vi "Begin.vi"(8 "error in":errorcluster) -> (0 "error out":errorcluster)   [LabVIEW 2016]
doc: "Called before other user functions, this VI is expected to open initial I/O refnums, load in file data, and do all program initialization. Notice that the <B>error out</B> terminal is simply used for data flow. Wiring it to other structures or subVIs ensures that this VI runs first."
uses:
  <vilib>/Rock Robotics/WPI/DriverStation/WPI_DriverStationRobotMode2.ctl
  <vilib>/Rock Robotics/SystemInterfaces/DIO/FPGA_DIOPWMChannel.ctl
  <vilib>/Rock Robotics/WPI/Joystick/WPI_JoystickDeviceEnum.ctl
  <vilib>/Rock Robotics/WPI/Solenoid/WPI_SolenoidChannel.ctl
  <vilib>/Rock Robotics/WPI/Camera/WPI_CameraExposure Values.ctl
  <vilib>/Rock Robotics/WPI/Camera/WPI_CameraWhite Balance Values.ctl
  <vilib>/Rock Robotics/WPI/Camera/WPI_CameraFrameRate.ctl
  <vilib>/Rock Robotics/WPI/Camera/WPI_CameraImageSize.ctl
  <vilib>/Rock Robotics/SystemInterfaces/DIO/FPGA_DIOChannel.ctl
  SubSystems/References/CameraDevRef 0.vi
  <vilib>/Rock Robotics/Network Tables/NT Write String Array.vi
  <vilib>/Rock Robotics/WPI/MotorControl/WPI_MotorControlOpen Talon.vi
  <vilib>/Rock Robotics/WPI/Solenoid/WPI_SolenoidOpenDouble.vi
  SubSystems/References/Refnums.vi
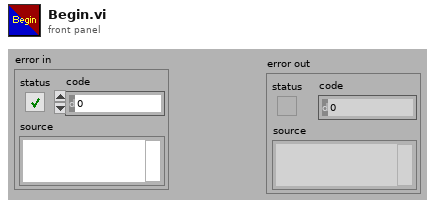
[diagram p1: front panel]
types:
  T1 = typedef "FPGA_DIOChannel.ctl" = enum8{"DIO 0", "DIO 1", "DIO 2", "DIO 3", "DIO 4", "DIO 5", "DIO 6", "DIO 7", "DIO 8", "DIO 9", "DIO MXP 0", "DIO MXP 1", "DIO MXP 2", "DIO MXP 3", "DIO MXP 4", "DIO MXP 5", "DIO MXP 6", "DIO MXP 7", "DIO MXP 8", "DIO MXP 9", "DIO MXP 10", "DIO MXP 11", "DIO MXP 12", "DIO MXP 13", "DIO MXP 14", "DIO MXP 15", "SPI Port CS1", "SPI Port CS2", "SPI Port CS3", "SPI Port MISO", "SPI Port MOSI", "Invalid"}
  T2 = typedef "WPI_CameraImageSize.ctl" = enum16{"640x480", "320x240", "160x120", "Custom"}
  T3 = typedef "WPI_CameraFrameRate.ctl" = u32
  T4 = typedef "WPI_CameraExposure Values.ctl" = enum16{"Auto", "Flicker-free 50 Hz", "Flicker-free 60 Hz", "Hold current", "Custom"}
  T5 = typedef "WPI_CameraWhite Balance Values.ctl" = enum16{"Auto", "Fixed indoor", "Fixed outdoor 1", "Fixed outdoor 2", "Fixed fluorescent 1", "Fixed fluorescent 2", "Hold current", "Custom"}
  T6 = typedef "FPGA_DIOPWMChannel.ctl" = enum8{"PWM 0", "PWM 1", "PWM 2", "PWM 3", "PWM 4", "PWM 5", "PWM 6", "PWM 7", "PWM 8", "PWM 9", "PWM MXP 0", "PWM MXP 1", "PWM MXP 2", "PWM MXP 3", "PWM MXP 4", "PWM MXP 5", "PWM MXP 6", "PWM MXP 7", "PWM MXP 8", "PWM MXP 9", "Invalid"}
  T7 = typedef "WPI_SolenoidChannel.ctl" = enum8{"Solenoid 0", "Solenoid 1", "Solenoid 2", "Solenoid 3", "Solenoid 4", "Solenoid 5", "Solenoid 6", "Solenoid 7", "Invalid"}
  T8 = typedef "WPI_JoystickDeviceEnum.ctl" = enum16{"USB 0", "USB 1", "USB 2", "USB 3", "USB 4", "USB 5"}
  T9 = typedef "WPI_DriverStationRobotMode2.ctl" = enum16{"Autonomous Disabled", "Autonomous Enabled", "Teleop Disabled", "Teleop Enabled", "Disconnected", "Finish", "Test Disabled", "Test Enabled", "Emergency Stopped"}
  T10 = typedef "WPI_CameraDevRef.ctl" = cluster{"Camera Address":string, "CameraStatus":errorcluster}
  T11 = typedef "WPI_JoystickDevRef.ctl" = cluster{"Device":T8}
  T12 = typedef "WPI_MotorControlDeviceRef.ctl" = cluster{"DeviceStatus":errorcluster, "Type":T13, "PWM":cluster{"PWM Channel":T6, "DeadBand":T14}, "CAN":cluster{"Device Number":u8, "SetOutput VI Ref":variant, "GetOutput VI Ref":variant, "Enable VI Ref":variant, "Disable VI Ref":variant, "Data":variant}, "Invert":bool}
  T13 = typedef "WPI_MotorControlType.ctl" = enum16{"PWM", "CAN"}
  T14 = typedef "WPI_PWMDeadband.ctl" = cluster{"Name":string, "maxPositivePwm":i32, "minPositivePwm":i32, "centerPwm":i32, "maxNegativePwm":i32, "minNegativePwm":i32, "angularRange":u16}
  T15 = typedef "WPI_DigitalInputDevRef.ctl" = cluster{"DevStatus":errorcluster, "DIO Channel":T1}
  T16 = typedef "WPI_SolenoidDevRef.ctl" = cluster{"DevStatus":errorcluster, "Pneumatics Control Module":u8, "Forward Solenoid Channel":T7, "Reverse Solenoid Channel":T7}
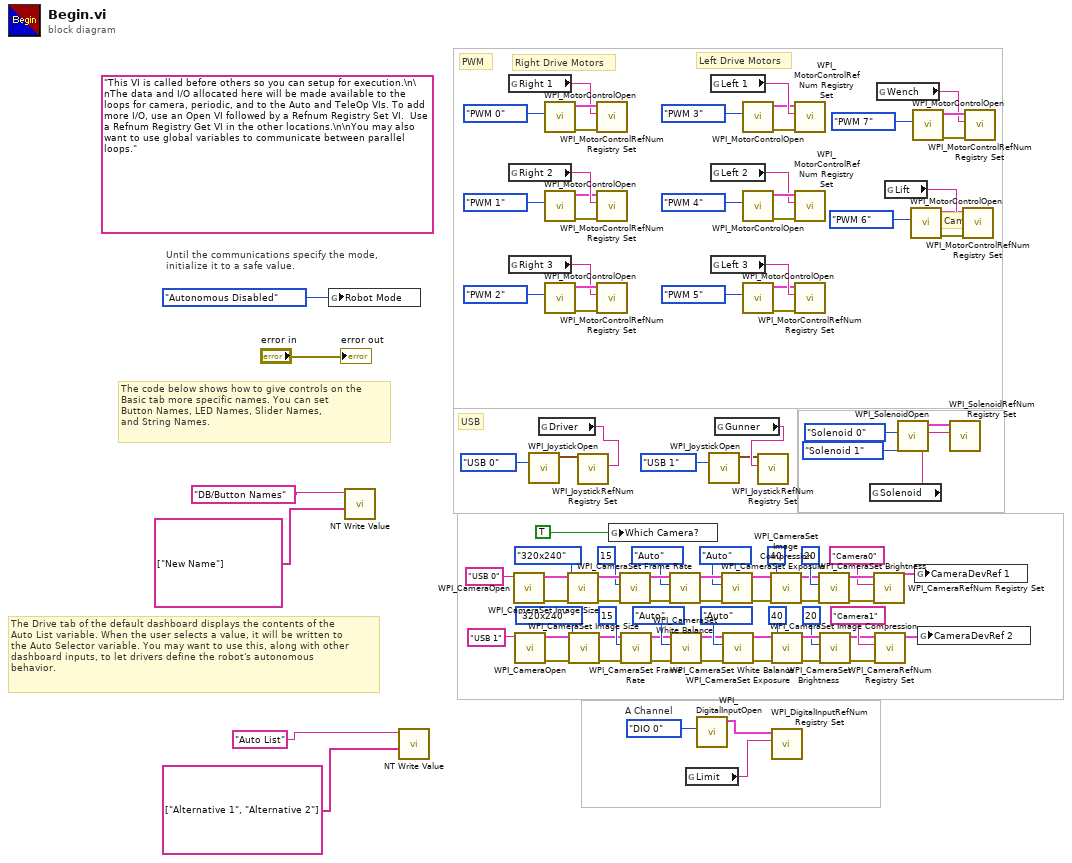
[diagram p0: block diagram]
diagram:
  w3 = FPGA_DIOChannel."DIO 0"  # A Channel
  (unwired) "This VI is called before others so you can setup for execution.\n\nThe data and I/O allocated here will be made available to the loops for camera, periodic, and to the Auto and TeleOp VIs. To add more I/O, use an Open VI followed by a Refnum Registry Set VI.  Use a Refnum Registry Get VI in the other locations.\n\nYou may also want to use global variables to communicate between parallel loops."
  # "Cameras"
  # "USB"
  # "Left Drive Motors"
  # "Right Drive Motors"
  # "PWM"
  # "The Drive tab of the default dashboard displays the contents of the\nAuto List variable. When the user selects a value, it will be written to\nthe Auto Selector variable. You may want to use this, along with other\ndashboard inputs, to let drivers define the robot's autonomous\nbehavior."
  # "The code below shows how to give controls on the\nBasic tab more specific names. You can set\nButton Names, LED Names, Slider Names,\nand String Names."
  # "Until the communications specify the mode,\ninitialize it to a safe value."
  n1 = global write "CameraDevRef 0.vi" "Robot Mode"(WPI_DriverStationRobotMode2."Autonomous Disabled" ("Robot Mode")) -> ()
  n2 = call-poly <vilib>:"NT Write Value.vi"("String Array"=string[] ["New Name"], "Name"="DB/Button Names") -> ()  [unwired: 9 in, 1 out]
  n3 = call-poly <vilib>:"NT Write Value.vi"("String Array"=string[] ["Alternative 1", "Alternative 2"], "Name"="Auto List") -> ()  [unwired: 9 in, 1 out]
  n4 = global read "Refnums.vi" "Right 1"() -> (w89:string)
  n5 = global read "Refnums.vi" "Right 2"() -> (w88:string)
  n6 = global read "Refnums.vi" "Right 3"() -> (w81:string)
  n7 = call <vilib>:"WPI_CameraOpen.vi"("Camera Address"="USB 0") -> ("error out"=w40:errorcluster, "CameraDevRef"=w41:T10)  [unwired: 1 in, 8 out]
  n8 = call <vilib>:"WPI_CameraOpen.vi"("Camera Address"="USB 1") -> ("error out"=w19:errorcluster, "CameraDevRef"=w18:T10)  [unwired: 1 in, 8 out]
  n9 = call <vilib>:"WPI_JoystickOpen.vi"("JoystickDevice"=WPI_JoystickDeviceEnum."USB 0") -> ("JoystickDevRef"=w64:T11)  [unwired: 10 in]
  n10 = global read "Refnums.vi" "Driver"() -> (w63:string)
  n11 = call-poly <vilib>:"WPI_MotorControlOpen.vi"("PWM Channel"=FPGA_DIOPWMChannel."PWM 0") -> ("error out"=w92:errorcluster, "MotorControlDeviceRef"=w91:T12)  [unwired: 9 in]
  n12 = call-poly <vilib>:"WPI_MotorControlOpen.vi"("PWM Channel"=FPGA_DIOPWMChannel."PWM 1") -> ("error out"=w85:errorcluster, "MotorControlDeviceRef"=w86:T12)  [unwired: 9 in]
  n13 = call-poly <vilib>:"WPI_MotorControlOpen.vi"("PWM Channel"=FPGA_DIOPWMChannel."PWM 2") -> ("error out"=w84:errorcluster, "MotorControlDeviceRef"=w83:T12)  [unwired: 9 in]
  n14 = call <vilib>:"WPI_CameraSet Image Size.vi"("error in (no error)"=w40, "Image Size"=WPI_CameraImageSize."320x240", "CameraDevRef"=w41) -> ("error out"=w39:errorcluster, "CameraDevRef Out"=w42:T10)  [unwired: 1 in, 6 out]
  n15 = call <vilib>:"WPI_CameraSet Image Size.vi"("error in (no error)"=w19, "Image Size"=WPI_CameraImageSize."320x240", "CameraDevRef"=w18) -> ("error out"=w20:errorcluster, "CameraDevRef Out"=w17:T10)  [unwired: 1 in, 6 out]
  n16 = call <vilib>:"WPI_JoystickRefNum Registry Set.vi"("refnum name"=w63, "JoystickDevRef"=w64) -> ()  [unwired: 8 in, 2 out]
  n17 = call <vilib>:"WPI_MotorControlRefNum Registry Set.vi"("error in (no error)"=w92, "refnum name"=w89, "MotorControlDevRef"=w91) -> ()  [unwired: 7 in, 2 out]
  n18 = call <vilib>:"WPI_MotorControlRefNum Registry Set.vi"("error in (no error)"=w85, "refnum name"=w88, "MotorControlDevRef"=w86) -> ()  [unwired: 7 in, 2 out]
  n19 = call <vilib>:"WPI_MotorControlRefNum Registry Set.vi"("error in (no error)"=w84, "refnum name"=w81, "MotorControlDevRef"=w83) -> ()  [unwired: 7 in, 2 out]
  n20 = global write "Refnums.vi" "Which Camera?"(TRUE ("Which Camera?")) -> ()
  n21 = call <vilib>:"WPI_CameraSet Frame Rate.vi"("error in (no error)"=w39, "Frame Rate (fps)"=T3 15, "CameraDevRef"=w42) -> ("error out"=w38:errorcluster, "CameraDevRef Out"=w44:T10)  [unwired: 7 out]
  n22 = call <vilib>:"WPI_CameraSet Frame Rate.vi"("error in (no error)"=w20, "Frame Rate (fps)"=T3 15, "CameraDevRef"=w17) -> ("error out"=w21:errorcluster, "CameraDevRef Out"=w15:T10)  [unwired: 7 out]
  n23 = call <vilib>:"WPI_CameraSet White Balance.vi"("error in (no error)"=w38, "White Balance"=WPI_CameraWhite_Balance_Values."Auto", "CameraDevRef"=w44) -> ("error out"=w37:errorcluster, "CameraDevRef Out"=w43:T10)  [unwired: 1 in, 6 out]
  n24 = call <vilib>:"WPI_CameraSet White Balance.vi"("error in (no error)"=w21, "White Balance"=WPI_CameraWhite_Balance_Values."Auto", "CameraDevRef"=w15) -> ("error out"=w22:errorcluster, "CameraDevRef Out"=w16:T10)  [unwired: 1 in, 6 out]
  n25 = global read "Refnums.vi" "Limit"() -> (w1:string)
  n26 = call <vilib>:"WPI_DigitalInputOpen.vi"("DIO Channel"=w3) -> ("DigitalInputDevRef"=w2:T15)  [unwired: 1 in, 9 out]
  n27 = call <vilib>:"WPI_JoystickOpen.vi"("JoystickDevice"=WPI_JoystickDeviceEnum."USB 1") -> ("JoystickDevRef"=w59:T11)  [unwired: 10 in]
  n28 = global read "Refnums.vi" "Left 1"() -> (w72:string)
  n29 = global read "Refnums.vi" "Left 2"() -> (w73:string)
  n30 = global read "Refnums.vi" "Left 3"() -> (w80:string)
  n31 = global read "Refnums.vi" "Gunner"() -> (w60:string)
  n32 = call <vilib>:"WPI_CameraSet Exposure.vi"("error in (no error)"=w37, "Exposure"=WPI_CameraExposure_Values."Auto", "CameraDevRef"=w43) -> ("error out"=w36:errorcluster, "CameraDevRef Out"=w46:T10)  [unwired: 1 in, 6 out]
  n33 = call <vilib>:"WPI_CameraSet Exposure.vi"("error in (no error)"=w22, "Exposure"=WPI_CameraExposure_Values."Auto", "CameraDevRef"=w16) -> ("error out"=w23:errorcluster, "CameraDevRef Out"=w13:T10)  [unwired: 1 in, 6 out]
  n34 = call-poly <vilib>:"WPI_MotorControlOpen.vi"("PWM Channel"=FPGA_DIOPWMChannel."PWM 3") -> ("error out"=w69:errorcluster, "MotorControlDeviceRef"=w70:T12)  [unwired: 9 in]
  n35 = call-poly <vilib>:"WPI_MotorControlOpen.vi"("PWM Channel"=FPGA_DIOPWMChannel."PWM 4") -> ("error out"=w76:errorcluster, "MotorControlDeviceRef"=w75:T12)  [unwired: 9 in]
  n36 = call-poly <vilib>:"WPI_MotorControlOpen.vi"("PWM Channel"=FPGA_DIOPWMChannel."PWM 5") -> ("error out"=w77:errorcluster, "MotorControlDeviceRef"=w78:T12)  [unwired: 9 in]
  n37 = call <vilib>:"WPI_JoystickRefNum Registry Set.vi"("refnum name"=w60, "JoystickDevRef"=w59) -> ()  [unwired: 8 in, 2 out]
  n38 = call <vilib>:"WPI_CameraSet Image Compression.vi"("error in (no error)"=w36, "Compression"=40, "CameraDevRef"=w46) -> ("error out"=w35:errorcluster, "CameraDevRef Out"=w45:T10)  [unwired: 7 out]
  n39 = call <vilib>:"WPI_CameraSet Image Compression.vi"("error in (no error)"=w23, "Compression"=40, "CameraDevRef"=w13) -> ("error out"=w24:errorcluster, "CameraDevRef Out"=w14:T10)  [unwired: 7 out]
  n40 = call <vilib>:"WPI_DigitalInputRefNum Registry Set.vi"("refnum name"=w1, "DigitalInputDevRef"=w2) -> ()  [unwired: 8 in, 2 out]
  n41 = call <vilib>:"WPI_MotorControlRefNum Registry Set.vi"("error in (no error)"=w69, "refnum name"=w72, "MotorControlDevRef"=w70) -> ()  [unwired: 7 in, 2 out]
  n42 = call <vilib>:"WPI_MotorControlRefNum Registry Set.vi"("error in (no error)"=w76, "refnum name"=w73, "MotorControlDevRef"=w75) -> ()  [unwired: 7 in, 2 out]
  n43 = call <vilib>:"WPI_MotorControlRefNum Registry Set.vi"("error in (no error)"=w77, "refnum name"=w80, "MotorControlDevRef"=w78) -> ()  [unwired: 7 in, 2 out]
  n44 = call <vilib>:"WPI_CameraSet Brightness.vi"("error in (no error)"=w35, "Brightness"=20, "CameraDevRef"=w45) -> ("error out"=w34:errorcluster, "CameraDevRef Out"=w50:T10)  [unwired: 7 out]
  n45 = call <vilib>:"WPI_CameraSet Brightness.vi"("error in (no error)"=w24, "Brightness"=20, "CameraDevRef"=w14) -> ("error out"=w25:errorcluster, "CameraDevRef Out"=w9:T10)  [unwired: 7 out]
  n46 = global read "Refnums.vi" "Solenoid"() -> (w57:string)
  n47 = call <vilib>:"WPI_CameraRefNum Registry Set.vi"("error in (no error)"=w34, "refnum name"="Camera0", "CameraDevRef"=w50) -> ("CameraDevRef"=w7:T10)  [unwired: 1 in, 7 out]
  n48 = call <vilib>:"WPI_CameraRefNum Registry Set.vi"("error in (no error)"=w25, "refnum name"="Camera1", "CameraDevRef"=w9) -> ("CameraDevRef"=w6:T10)  [unwired: 1 in, 7 out]
  n49 = global read "Refnums.vi" "Wench"() -> (w65:string)
  n50 = global read "Refnums.vi" "Lift"() -> (w54:string)
  n51 = call-poly <vilib>:"WPI_SolenoidOpen.vi"("Reverse Solenoid Channel"=WPI_SolenoidChannel."Solenoid 1", "Forward Solenoid Channel"=WPI_SolenoidChannel."Solenoid 0" ("Solenoid Channel")) -> ("SolenoidDevRef"=w58:T16)  [unwired: 8 in, 1 out]
  n52 = call-poly <vilib>:"WPI_MotorControlOpen.vi"("PWM Channel"=FPGA_DIOPWMChannel."PWM 6") -> ("error out"=w51:errorcluster, "MotorControlDeviceRef"=w52:T12)  [unwired: 9 in]
  n53 = call-poly <vilib>:"WPI_MotorControlOpen.vi"("PWM Channel"=FPGA_DIOPWMChannel."PWM 7") -> ("error out"=w68:errorcluster, "MotorControlDeviceRef"=w67:T12)  [unwired: 9 in]
  n54 = global write "Refnums.vi" "CameraDevRef 1"(w7) -> ()
  n55 = global write "Refnums.vi" "CameraDevRef 2"(w6) -> ()
  n56 = call <vilib>:"WPI_SolenoidRefNum Registry Set.vi"("refnum name"=w57, "SolenoidDevRef"=w58) -> ()  [unwired: 8 in, 2 out]
  n57 = call <vilib>:"WPI_MotorControlRefNum Registry Set.vi"("error in (no error)"=w51, "refnum name"=w54, "MotorControlDevRef"=w52) -> ()  [unwired: 7 in, 2 out]
  n58 = call <vilib>:"WPI_MotorControlRefNum Registry Set.vi"("error in (no error)"=w68, "refnum name"=w65, "MotorControlDevRef"=w67) -> ()  [unwired: 7 in, 2 out]
  "error out" <- "error in"
